vi "FTW-Tree-GetChildNodes.vi"(0 "Tree Ctl Ref":refnum<vi>, 5 "Parent Tag":string, 7 "Regex Filter (blank to return all children)":string, 11 "error in":errorcluster) -> (4 "Tree Ctl Ref out":refnum<vi>, 6 "Matching Child Node Tags":string[](array[string]), 15 "error out":errorcluster)   [LabVIEW 2014]
panel:
  # "Inputs"
  # "Outputs"
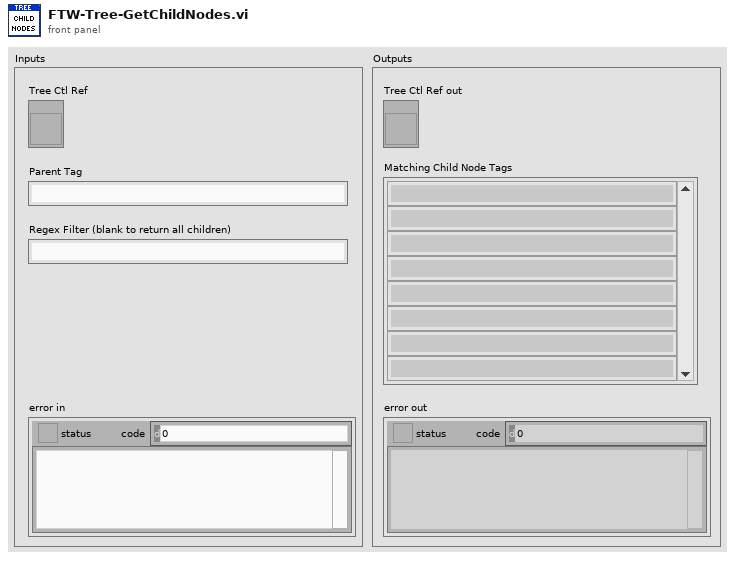
[diagram p1: front panel]
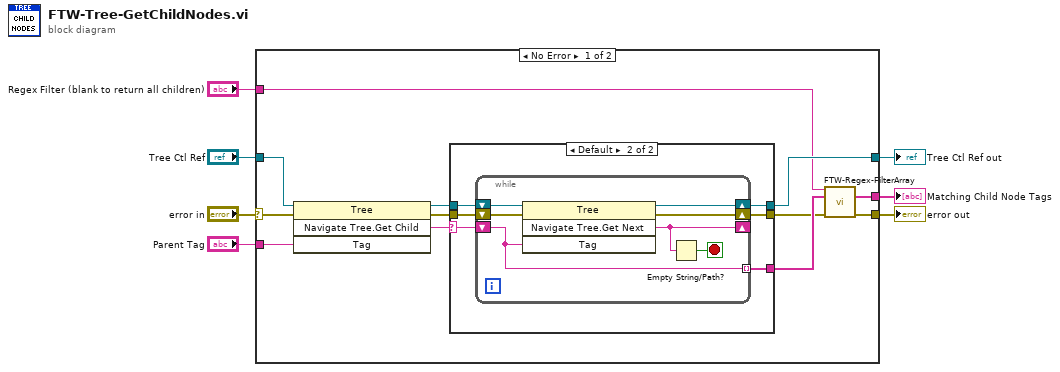
[diagram p0: block diagram]
diagram:
  n1 = case shown="No Error" "error in" {
    selector: "error in" -> [w19 w36]
    tunnel: [w10 w36] -> w7
    tunnel: "Tree Ctl Ref" -> [w18 w35]
    tunnel: "Parent Tag" -> [w17 _]
    tunnel: [w13 w35] -> w4
    tunnel: [w11 _] -> w2
    tunnel: "Regex Filter (blank to return all children)" -> [w8 _]
    frame No Error {
      n2 = invoke class="Tree" method="Navigate Tree.Get Child"(reference=w18, error in=w19, "Tag"=w17) -> (reference out=w15:refnum<vi>, error out=w14:errorcluster, "Navigate Tree:Get Child"=w16:string)  [unwired: 1 in, 1 out]
      n3 = case shown="Default" w16 {
        selector: w16 -> [_ w24]
        tunnel: w15 -> [w21 w27]
        tunnel: w14 -> [w20 w26]
        tunnel: [w21 w25] -> w13
        tunnel: [w20 w23] -> w9
        tunnel: [_ w22] -> w12
        frame "" {
        }
        frame Default {
          n4 = while {
            shift-right: [w32] -> w25
            shift-left: w27 -> [w34]
            shift-right: [w30] -> _
            shift-left: w24 -> [w28]
            shift-right: [w31] -> w23
            shift-left: w26 -> [w33]
            tunnel: [w28] -> w22 mode=indexing
            stop <- w29 stop-if-true
            n5 = invoke class="Tree" method="Navigate Tree.Get Next"(reference=w34, error in=w33, "Tag"=w28) -> (reference out=w32:refnum<vi>, error out=w31:errorcluster, "Navigate Tree:Get Next Item"=w30:string)  [unwired: 1 in, 1 out]
            n6 = Empty String/Path?(string/path=w30) -> (empty?=w29:bool)
          }
        }
      }
      n7 = call "FTW-Regex-FilterArray.vi"("Regex Filter"=w8, "Input Array"=w12, "error in"=w9) -> ("Matching Items"=w11:string[], "error out"=w10:errorcluster)  [unwired: 10 in, 1 out]
    }
    frame Error {
    }
  }
  "error out" <- w7
  "Tree Ctl Ref out" <- w4
  "Matching Child Node Tags" <- w2
